vi "StartVI.vi"(11 "error in":errorcluster) -> (4 "Application Ref out":refnum<vi>, 6 "VI Reference":refnum<vi>, 15 "error out":errorcluster)   [LabVIEW 2016, in "CarWashTest.lvlib"]
doc: "Run the main VI"
uses:
  CarWashTest.lvlib
  Drona.lvlib
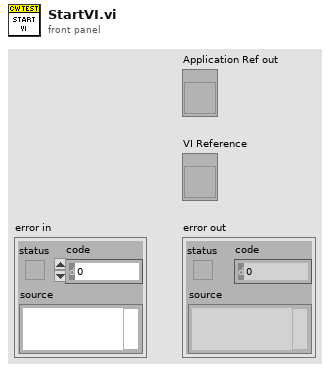
[diagram p1: front panel]
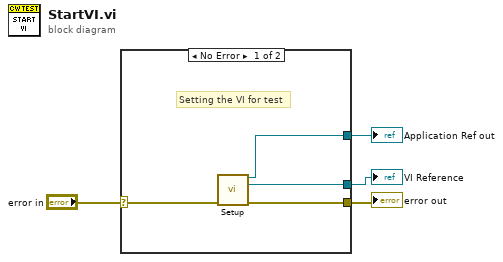
[diagram p0: block diagram]
diagram:
  n1 = case shown="No Error" "error in" {
    selector: "error in" -> [w8 w9]
    tunnel: [w7 _] -> w3
    tunnel: [w6 _] -> w2
    tunnel: [w5 w9] -> w1
    frame No Error {
      # "Setting the VI for test"
      n2 = call "Setup.vi"("error in"=w8) -> ("Application Ref"=w7:refnum<vi>, "VI Reference Out"=w6:refnum<vi>, "error out"=w5:errorcluster)  [unwired: 12 in]
    }
    frame Error {
    }
  }
  "Application Ref out" <- w3
  "VI Reference" <- w2
  "error out" <- w1
